vi "Post-Build Action_Make copy for LV2015.vi"(5 "Files Generated by Build":path[](array[path]), 6 "Top Level/Always Included VIs":path[](array[path]), 7 "Destination Path":path, 8 "error in (no error)":errorcluster, 9 "Target Name":string, 10 "Build Specification Name":string, 11 "Project Path":path) -> (0 "error out":errorcluster)   [LabVIEW 2023]
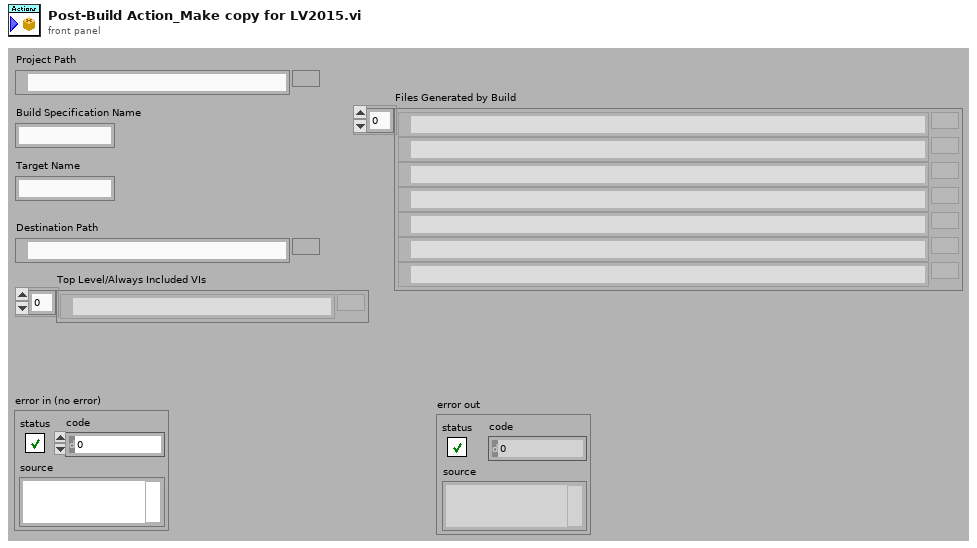
[diagram p1: front panel]
types:
  T1 = enum16{"Stop on First Error and report", "Continue on Error and Report", "Clear all Errors"}
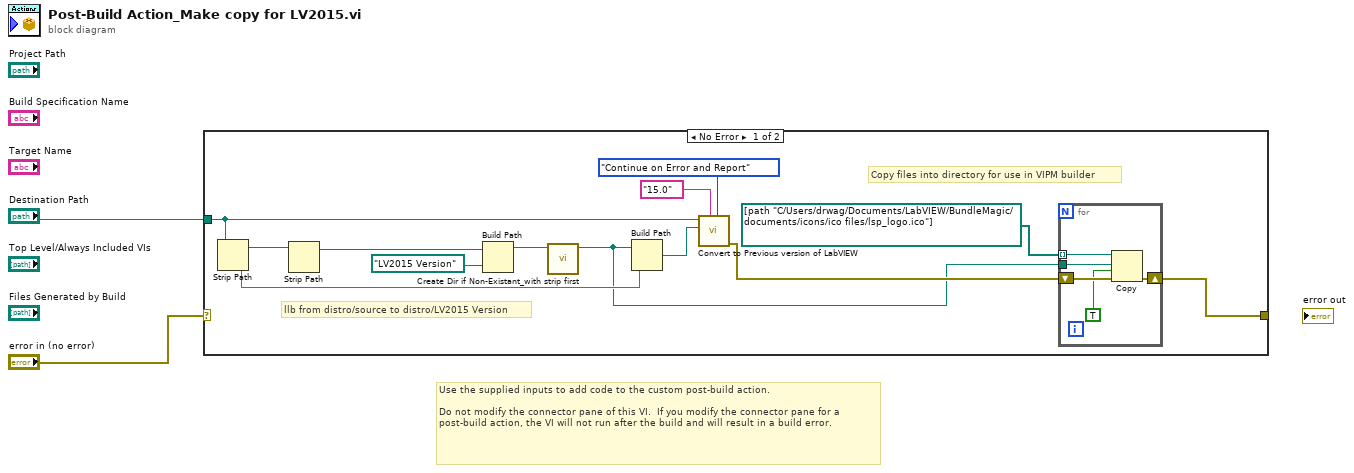
[diagram p0: block diagram]
diagram:
  # "Use the supplied inputs to add code to the custom post-build action.\n\nDo not modify the connector pane of this VI.  If you modify the connector pane for a post-build action, the VI will not run after the build and will result in a build error."
  n1 = case shown="No Error" "error in (no error)" {
    selector: "error in (no error)" -> [_ w21]
    tunnel: "Destination Path" -> [w7 _]
    tunnel: [w8 w21] -> _
    frame No Error {
      # "llb from distro/source to distro/LV2015 Version"
      # "Copy files into directory for use in VIPM builder"
      n2 = Strip Path(path=w7) -> (stripped path=w4:path, name=w13:string)
      n3 = Strip Path(path=w4) -> (stripped path=w3:path)  [unwired: 1 out]
      n4 = Build Path(base path=w3, name or relative path=path "LV2015 Version") -> (appended path=w6:path)
      n5 = call "Create Dir if Non-Existant_with strip first.vi"("Directory Path"=w6) -> ("dup Directory Path"=w5:path)  [unwired: 8 in, 2 out]
      n6 = Build Path(base path=w5, name or relative path=w13) -> (appended path=w10:path)
      n7 = call "Convert to Previous version of LabVIEW.vi"("Error Handling"=T1."Continue on Error and Report", "Previous Version"="15.0", "Destination for down converted files."=w10, "Folder of LabVIEW files"=w7) -> ("error out"=w11:errorcluster)  [unwired: 6 in, 1 out]
      n8 = for {
        shift-right: [w19] -> w8
        shift-left: w11 -> [w20]
        tunnel: path[] [path "C:/Users/drwag/Documents/LabVIEW/BundleMagic/documents/icons/ico files/lsp_logo.ico"] ("name or relative path") -> [w18] mode=indexing
        tunnel: w5 -> [w17]
        n9 = Copy(8:w20, 9:TRUE ("overwrite (F)"), 10:w17, 11:w18) -> (0:w19:errorcluster)  [unwired: 1 in, 2 out]
      }
    }
    frame Error {
    }
  }
